vi "Game_Setting.vi"(10 "true":bool, 11 "Difficulty":enum16{"Easy", "Medium", "Hard"}(ring)) -> (1 "milliseconds to wait":u32, 2 "Num of Circles":i32, 3 "radius 2":i16, 4 "radius":i16)   [LabVIEW 2021]
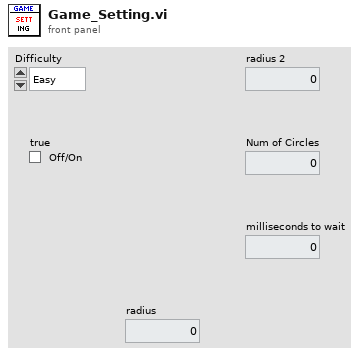
[diagram p1: front panel]
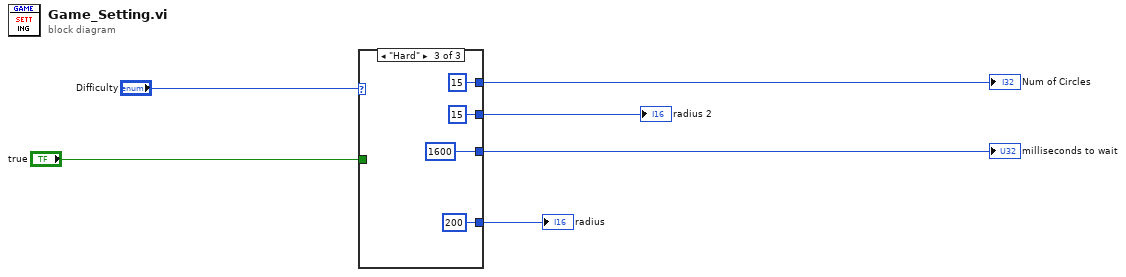
[diagram p0: block diagram]
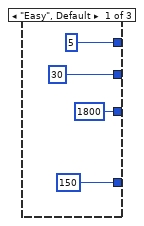
[diagram p2: hidden frame]
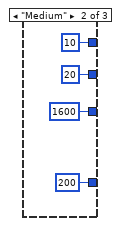
[diagram p3: hidden frame]
diagram:
  n1 = case shown="\"Hard\"" "Difficulty" {
    tunnel: [5 10 15] -> w1
    tunnel: [i16 30 ("radius") i16 20 ("radius") i16 15 ("radius")] -> w3
    tunnel: [u32 1800 ("milliseconds to wait") u32 1600 ("milliseconds to wait") u32 1600 ("milliseconds to wait")] -> w2
    tunnel: [i16 150 ("radius") i16 200 ("radius") i16 200 ("radius")] -> w4
    tunnel: "true" -> [_ _ _]
    frame "Easy", Default {
    }
    frame "Medium" {
    }
    frame "Hard" {
    }
  }
  "radius" <- w4
  "radius 2" <- w3
  "milliseconds to wait" <- w2
  "Num of Circles" <- w1
